vi "Robot Global Data.vi"() -> ()   [LabVIEW 2020]
doc: "This global VI can contain as many global variables as you need. Place a control on the panel, give it a good name. To read or write to it from a VI, drag the icon to the diagram of that VI. You can also drag from the project. Click on the node to change which global you access. You shouldn't have multiple locations writing to a global or it will cause a race-condition."
uses:
  <vilib>/Rock Robotics/WPI/Camera/WPI_CameraImageSize.ctl
  <vilib>/Rock Robotics/WPI/DriverStation/WPI_DriverStationRobotMode2.ctl
panel:
  out "Right Trigger":bool
  out "Left Trigger":bool
  out "Drive Mode":dbl
  out "Fancy Swerve":bool
  out "Fast Launch T-Shirt?":bool
  out "Medium Launch T-Shirt?":bool
  in  "Dart Speed":dbl
  in  "Right Joystick Y":dbl
  in  "# of the Dart":i32
  out "Dart Potentiometer Actual Value":dbl
  out "Dart #2":T1
  out "Pusher State":string
  out "Push T-Shirt?":bool
  out "Pusher Angle":dbl
  out "Push T-Shirt Start?":bool
  in  "Back Left Pivot Motor Wanted Angle":dbl
  in  "Back Left Pivot Motor Current Angle":dbl
  in  "Back Left Drive Motor Speed":dbl
  in  "Right Joystick X":dbl
  out "Center Spin Latch":bool
  in  "Back Right Pivot Motor Wanted Angle":dbl
  in  "Back Right Pivot Motor Current Angle":dbl
  in  "Back Right Drive Motor Speed":dbl
  in  "Front Left Pivot Motor Wanted Angle":dbl
  in  "Front Left Pivot Motor Current Angle":dbl
  in  "Front Left Drive Motor Speed":dbl
  out "Optical Encoder Wanted Count":dbl
  out "Optical Encoder Current Count":dbl
  out "Rotate Chamber?":bool
  out "Rotate Chamber Start?":bool
  in  "Left Joystick Y":dbl
  in  "Left Joystick X":dbl
  in  "Front Right Pivot Motor Wanted Angle":dbl
  in  "Front Right Pivot Motor Current Angle":dbl
  in  "Front Right Drive Motor Speed":dbl
  out "Slow Launch T-Shirt?":bool
  out "Right Big Launcher Encoder Velocity":dbl
  out "Left Big Launcher Encoder Velocity":dbl
  in  "Robot Mode":T2
  in  "image size":T3=enum."320x240"
  in  "Enable Vision":bool
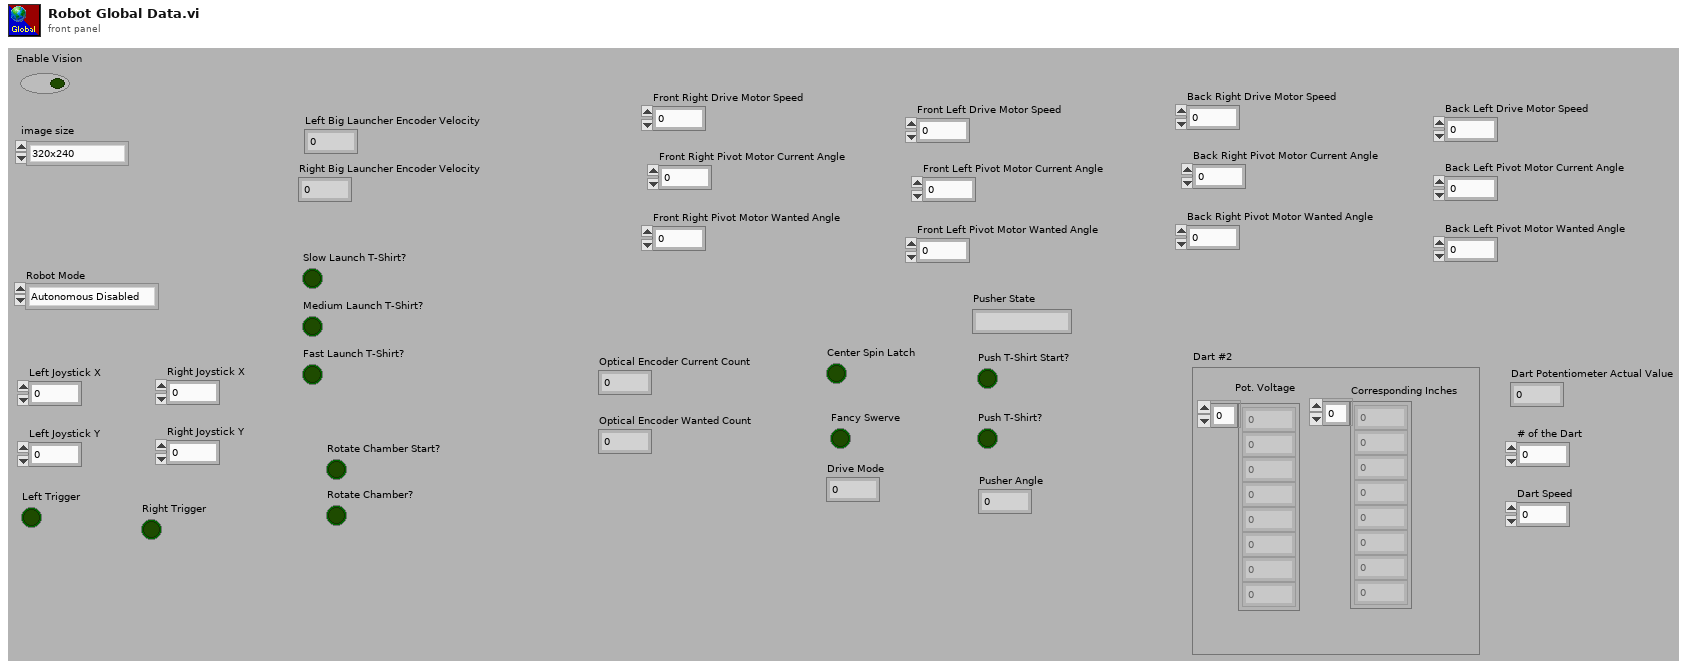
[diagram p1: front panel]
types:
  T1 = cluster{"Pot. Voltage":dbl[], "Corresponding Inches":dbl[]}
  T2 = typedef "WPI_DriverStationRobotMode2.ctl" = enum16{"Autonomous Disabled", "Autonomous Enabled", "Teleop Disabled", "Teleop Enabled", "Disconnected", "Finish", "Test Disabled", "Test Enabled", "Emergency Stopped"}
  T3 = typedef "WPI_CameraImageSize.ctl" = enum16{"640x480", "320x240", "160x120", "Custom"}
diagram:
